vi "Section parameter check.vi"(8 "error in":errorcluster, 9 "Row number":u32, 10 "Tbl Refnum in":refnum<vi>, 11 "Tree Refnum in":refnum<vi>) -> (0 "error out":errorcluster, 1 "Check result":string="√", 2 "Tbl Refnum out":refnum<vi>, 3 "Tree Refnum out":refnum<vi>)   [LabVIEW 2010]
panel:
  out "Enum":T1(ring)=enum."float"
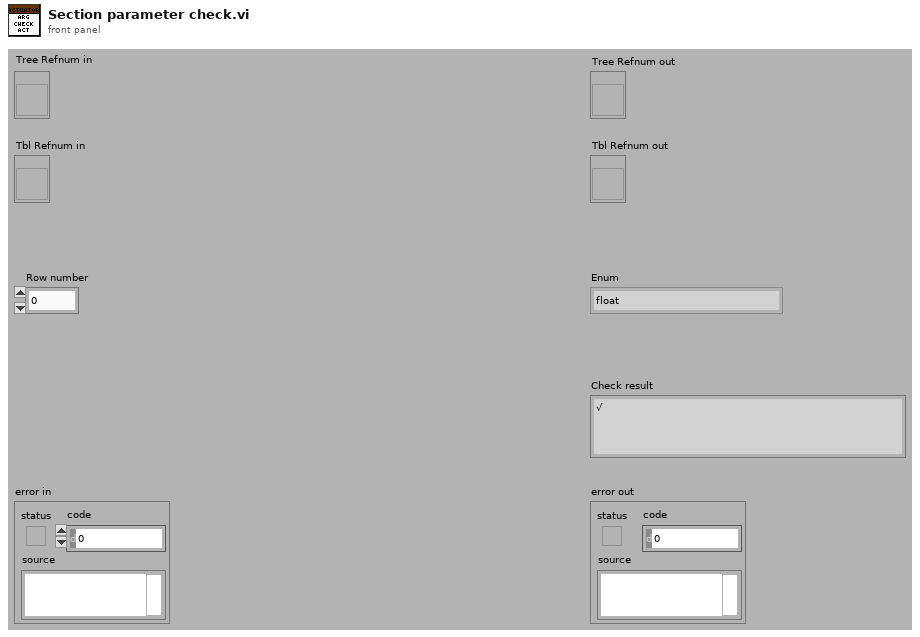
[diagram p1: front panel]
types:
  T1 = enum16{"char", "float", "double", "int", "long", "qword", "enum"}
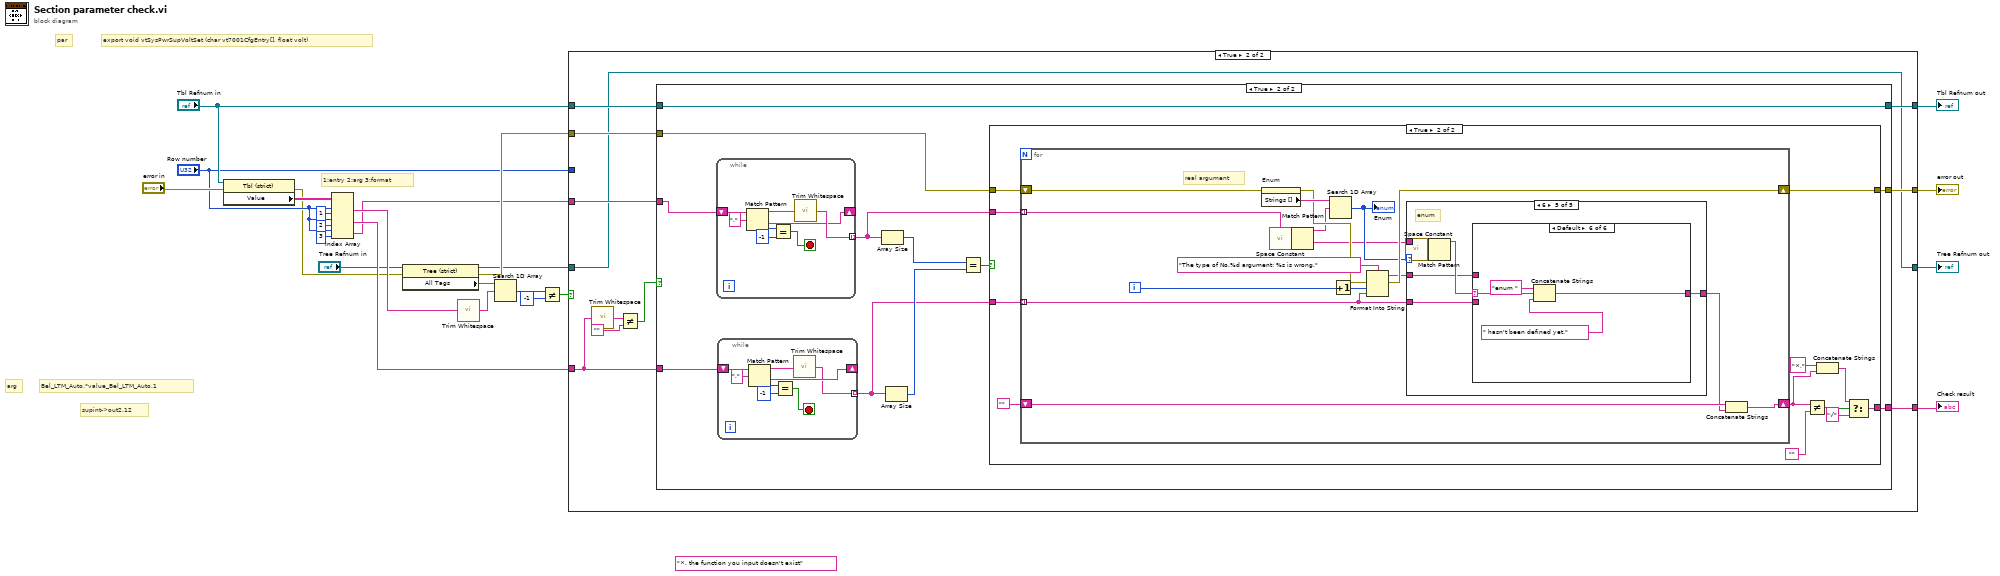
[diagram p0: block diagram]
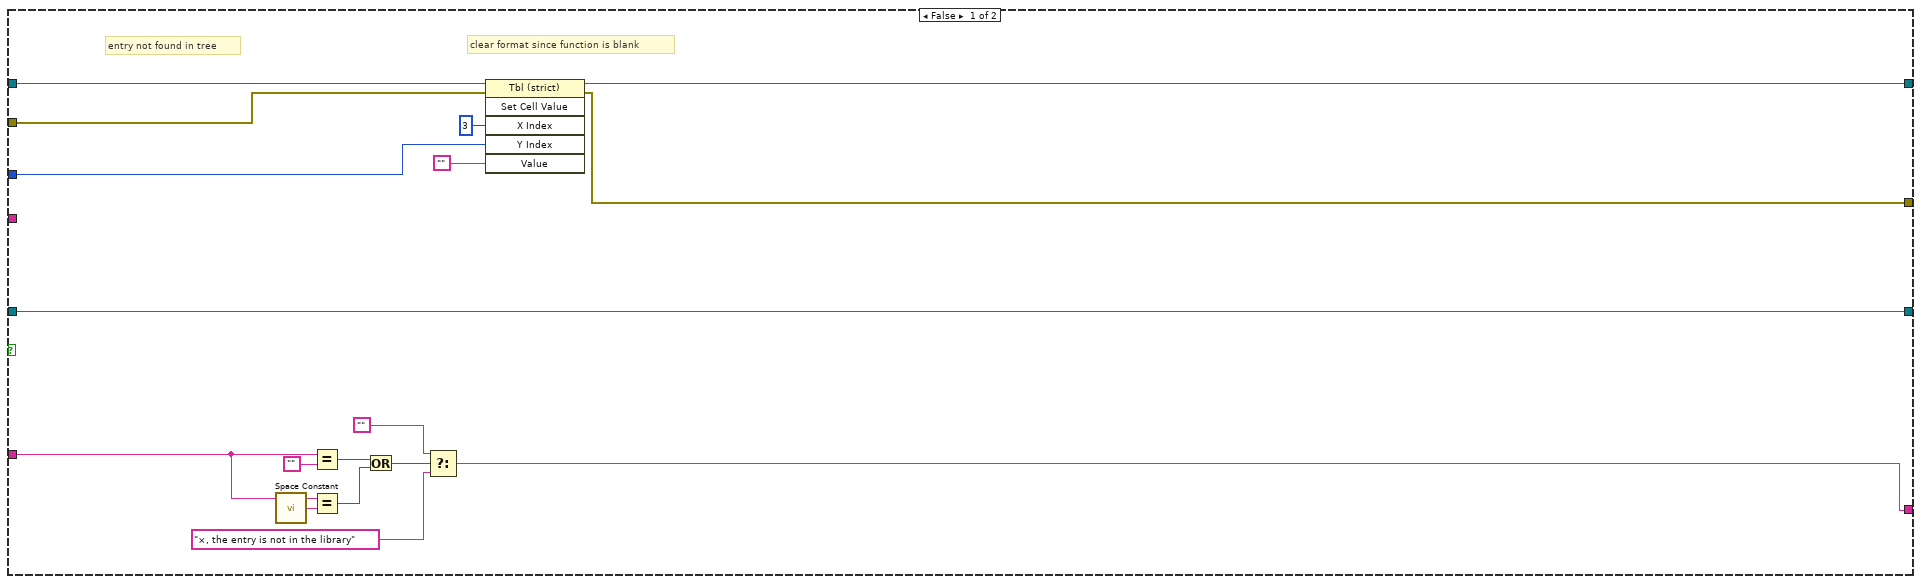
[diagram p2: hidden frame]
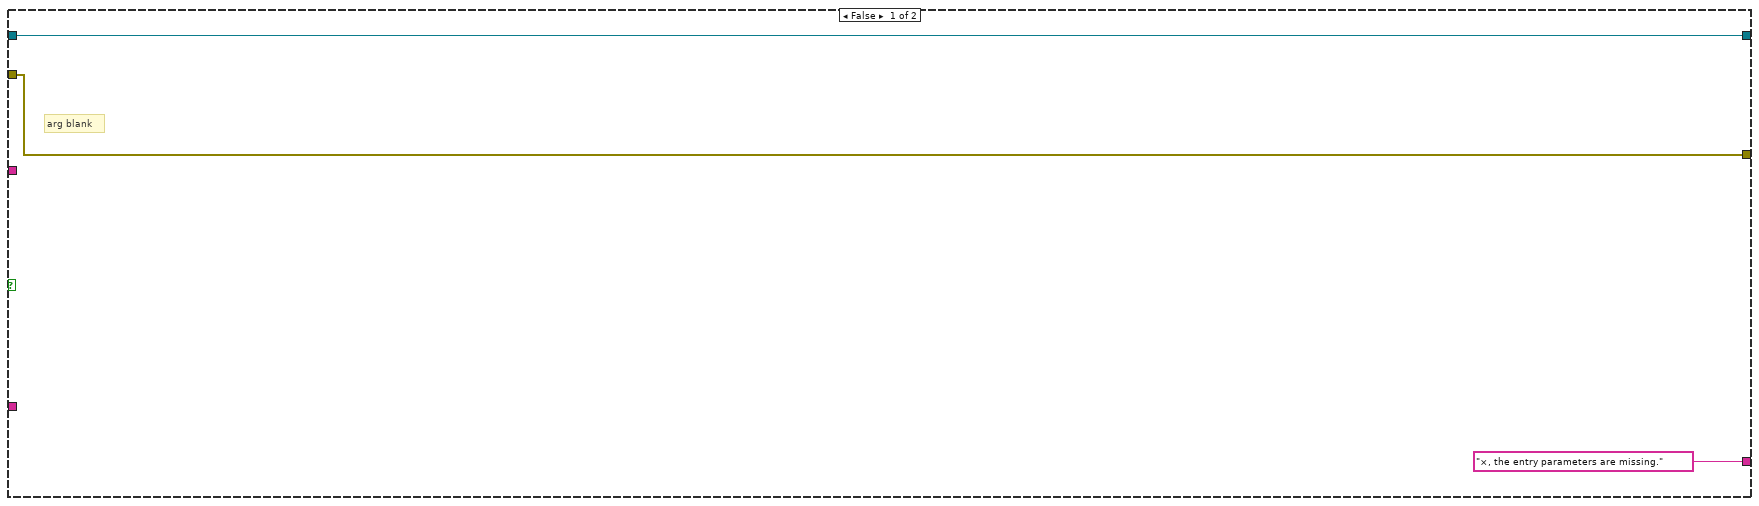
[diagram p3: hidden frame]
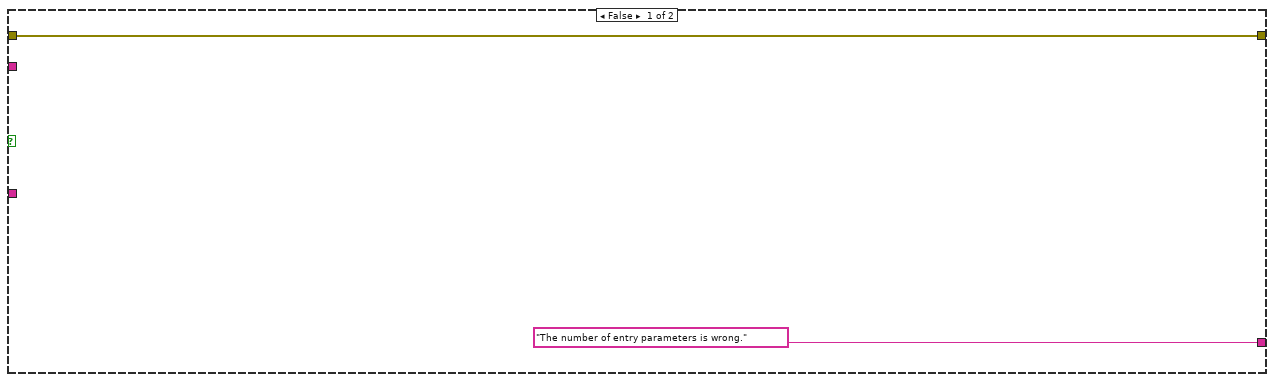
[diagram p4: hidden frame]
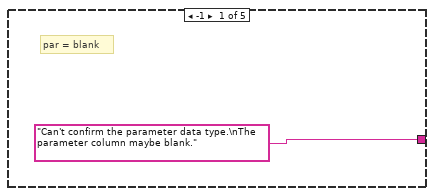
[diagram p5: hidden frame]
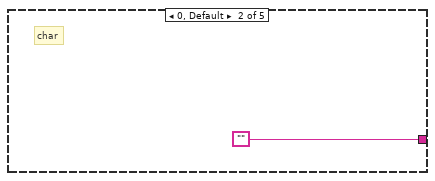
[diagram p6: hidden frame]
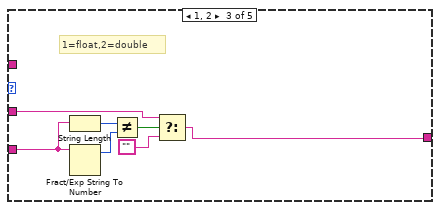
[diagram p7: hidden frame]
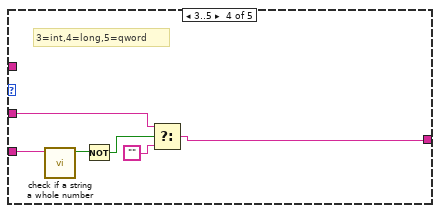
[diagram p8: hidden frame]
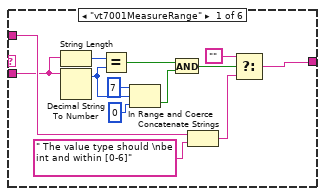
[diagram p9: hidden frame]
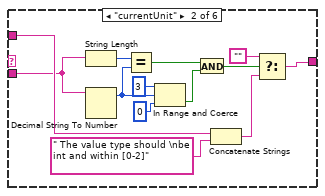
[diagram p10: hidden frame]
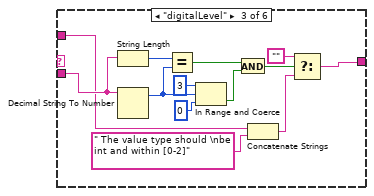
[diagram p11: hidden frame]
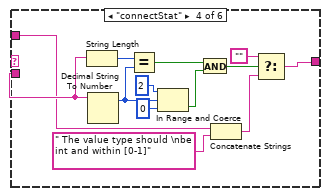
[diagram p12: hidden frame]
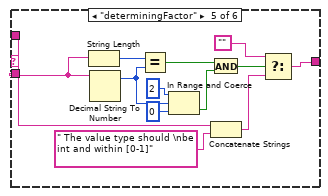
[diagram p13: hidden frame]
diagram:
  (unwired) "×, the function you input doesn't exist" ("Value")
  # "arg"
  # "par"
  # "1:entry 2:arg 3:format"
  # "Bel_LTM_Auto,*value_Bel_LTM_Auto,1"
  # "supint->out2,12"
  # "export void vtSysPwrSupVoltSet (char vt7001CfgEntry[], float volt)"
  n1 = property class="Tbl (strict)"(reference="Tbl Refnum in", error in="error in") -> (error out=w1:errorcluster, "Value"=w11:string[][])  [unwired: 1 out]
  n2 = Index Array(array=w11, index (row) #1="Row number", index (col) #1=1 ("disabled index (col)"), index (row) #2="Row number", index (col) #2=2 ("index (col)"), index (row) #3="Row number", index (col) #3=3 ("disabled index (col)")) -> (element #1=w5:string, element #2=w4:string, element #3=w3:string)
  n3 = property on="Property Node" class="Tree (strict)"(reference="Tree Refnum in", error in=w1) -> (reference out=w14:refnum<vi>, error out=w15:errorcluster, "All Tags"=w19:string[])
  n4 = call <vilib>:"Trim Whitespace.vi"("string"=w5) -> ("trimmed string"=w18:string)  [unwired: 1 in]
  n5 = Search 1D Array(1D array=w19, element=w18) -> (index of element=w17:i32)  [unwired: 1 in]
  n6 = Not Equal?(x=w17, y=-1) -> (x != y?=w23:bool)
  n7 = case shown="True" w23 {
    tunnel: w3 -> [_ w51]
    tunnel: w4 -> [w30 w42]
    tunnel: w15 -> [w33 w50]
    tunnel: [w24 w49] -> w22
    tunnel: [w37 w48] -> w21
    tunnel: "Tbl Refnum in" -> [w34 w47]
    tunnel: "Row number" -> [w35 _]
    tunnel: [w38 w46] -> w20
    tunnel: w14 -> [w36 w41]
    tunnel: [w36 w41] -> w13
    frame False {
      # "clear format since function is blank"
      # "entry not found in tree"
      n8 = call <vilib>:"Space Constant.vi"() -> ("String"=w31:string)
      n9 = Equal?(x=w30, y="") -> (x = y?=w29:bool)
      n10 = Equal?(x=w30, y=w31) -> (x = y?=w28:bool)
      n11 = Or(x=w29, y=w28) -> (x .or. y?=w27:bool)
      n12 = Select(t="", s=w27, f="×, the entry is not in the library") -> (s? t:f=w24:string)
      n13 = invoke class="Tbl (strict)" method="Set Cell Value"(reference=w34, error in=w33, "X Index"=u32 3, "Y Index"=w35, "Value"="") -> (reference out=w38:refnum<vi>, error out=w37:errorcluster)  [unwired: 1 in, 4 out]
    }
    frame True {
      n14 = call <vilib>:"Trim Whitespace.vi"("string"=w42) -> ("trimmed string"=w45:string)  [unwired: 1 in]
      n15 = Not Equal?(x=w45, y="") -> (x != y?=w43:bool)
      n16 = case shown="True" w43 {
        tunnel: w51 -> [_ w55]
        tunnel: w42 -> [_ w60]
        tunnel: w50 -> [w53 w59]
        tunnel: ["×, the entry parameters are missing." w58] -> w49
        tunnel: [w53 w57] -> w48
        tunnel: w47 -> [w54 w56]
        tunnel: [w54 w56] -> w46
        frame False {
          # "arg blank"
        }
        frame True {
          n17 = while {
            shift-right: [w195] -> _
            shift-left: w55 -> [w202]
            tunnel: [w196] -> w62 mode=indexing
            stop <- w198 stop-if-true
            n18 = Match Pattern(string=w202, regular expression=",") -> (before substring=w197:string, after substring=w195:string, offset past match=w200:i32)  [unwired: 1 in, 1 out]
            n19 = Equal?(x=w200, y=-1) -> (x = y?=w198:bool)
            n20 = call <vilib>:"Trim Whitespace.vi"("string"=w197) -> ("trimmed string"=w196:string)  [unwired: 1 in]
          }
          n21 = while {
            shift-right: [w190] -> _
            shift-left: w60 -> [w194]
            tunnel: [w187] -> w61 mode=indexing
            stop <- w189 stop-if-true
            n22 = Match Pattern(string=w194, regular expression=",") -> (before substring=w188:string, after substring=w190:string, offset past match=w192:i32)  [unwired: 1 in, 1 out]
            n23 = Equal?(x=w192, y=-1) -> (x = y?=w189:bool)
            n24 = call <vilib>:"Trim Whitespace.vi"("string"=w188) -> ("trimmed string"=w187:string)  [unwired: 1 in]
          }
          n25 = Array Size(array=w62) -> (size(s)=w65:i32)
          n26 = Array Size(array=w61) -> (size(s)=w64:i32)
          n27 = Equal?(x=w65, y=w64) -> (x = y?=w63:bool)
          n28 = case shown="True" w63 {
            tunnel: w62 -> [_ w79]
            tunnel: w61 -> [_ w78]
            tunnel: ["The number of entry parameters is wrong." w73] -> w58
            tunnel: w59 -> [w66 w72]
            tunnel: [w66 w71] -> w57
            frame False {
            }
            frame True {
              n29 = for {
                tunnel: w79 -> [w80] mode=indexing
                tunnel: w78 -> [w91] mode=indexing
                shift-right: [w95] -> w69
                shift-left: "" -> [w96]
                shift-right: [w93] -> w71
                shift-left: w72 -> [w94]
                i -> [w92]
                # "real argument"
                n30 = property on="Enum" class="Enum (strict)"(error in=w94) -> (error out=w85:errorcluster, "Strings []"=w89:string[])  [unwired: 1 in, 1 out]
                n31 = call <vilib>:"Space Constant.vi"() -> ("String"=w90:string)
                n32 = Match Pattern(string=w80, regular expression=w90) -> (before substring=w82:string, after substring=w81:string)  [unwired: 1 in, 2 out]
                n33 = Search 1D Array(1D array=w89, element=w82) -> (index of element=w88:i32)  [unwired: 1 in]
                "Enum" <- w88
                n34 = Increment(x=w92) -> (x+1=w86:i32)
                n35 = Format Into String(format string="The type of No.%d argument: %s is wrong.", error in=w85, w86, w91) -> (resulting string=w84:string, error out=w93:errorcluster)  [unwired: 1 in]
                n36 = case shown="6" w88 {
                  tunnel: w91 -> [_ _ w103 w108 w113]
                  tunnel: w84 -> [_ _ w100 w111 w114]
                  tunnel: ["Can't confirm the parameter data type.\nThe parameter column maybe blank." "" w99 w109 w112] -> w83
                  tunnel: w81 -> [_ _ _ _ w117]
                  frame -1 {
                    # "par = blank"
                  }
                  frame 0, Default {
                    # "char"
                  }
                  frame 1, 2 {
                    # "1=float,2=double"
                    n37 = String Length(string=w103) -> (length=w105:i32)
                    n38 = Fract/Exp String To Number(string=w103) -> (offset past number=w104:i32)  [unwired: 3 in, 1 out]
                    n39 = Not Equal?(x=w105, y=w104) -> (x != y?=w102:bool)
                    n40 = Select(t=w100, s=w102, f="") -> (s? t:f=w99:string)
                  }
                  frame 3..5 {
                    # "3=int,4=long,5=qword"
                    n41 = call "check if a string a whole number.vi"("input string"=w108) -> ("is a whole number?"=w107:bool)  [unwired: 10 in]
                    n42 = Not(x=w107) -> (.not. x?=w106:bool)
                    n43 = Select(t=w111, s=w106, f="") -> (s? t:f=w109:string)
                  }
                  frame 6 {
                    # "enum"
                    n44 = call <vilib>:"Space Constant.vi"() -> ("String"=w116:string)
                    n45 = Match Pattern(string=w117, regular expression=w116) -> (before substring=w115:string)  [unwired: 1 in, 3 out]
                    n46 = case shown="Default" w115 {
                      selector: w115 -> [_ _ _ _ _ w186]
                      tunnel: w114 -> [w120 w133 w145 w158 w171 _]
                      tunnel: w113 -> [w119 w132 w146 w159 w173 _]
                      tunnel: [w118 w131 w144 w157 w172 w184] -> w112
                      frame "vt7001MeasureRange" {
                        n47 = String Length(string=w119) -> (length=w130:i32)
                        n48 = Decimal String To Number(string=w119) -> (offset past number=w128:i32)  [unwired: 2 in, 1 out]
                        n49 = Equal?(x=w130, y=w128) -> (x = y?=w129:bool)
                        n50 = In Range and Coerce(upper limit=7, x=w128, lower limit=0) -> (In Range?=w125:bool)  [unwired: 1 out]
                        n51 = And(x=w129, y=w125) -> (x .and. y?=w124:bool)
                        n52 = Concatenate Strings(w120, " The value type should \nbe int and within [0-6]" ("string")) -> (w122:string)
                        n53 = Select(t="", s=w124, f=w122) -> (s? t:f=w118:string)
                      }
                      frame "currentUnit" {
                        n54 = String Length(string=w132) -> (length=w143:i32)
                        n55 = Decimal String To Number(string=w132) -> (offset past number=w141:i32)  [unwired: 2 in, 1 out]
                        n56 = Equal?(x=w143, y=w141) -> (x = y?=w142:bool)
                        n57 = In Range and Coerce(upper limit=3, x=w141, lower limit=0) -> (In Range?=w138:bool)  [unwired: 1 out]
                        n58 = And(x=w142, y=w138) -> (x .and. y?=w137:bool)
                        n59 = Concatenate Strings(w133, " The value type should \nbe int and within [0-2]" ("string")) -> (w135:string)
                        n60 = Select(t="", s=w137, f=w135) -> (s? t:f=w131:string)
                      }
                      frame "digitalLevel" {
                        n61 = String Length(string=w146) -> (length=w156:i32)
                        n62 = Decimal String To Number(string=w146) -> (offset past number=w154:i32)  [unwired: 2 in, 1 out]
                        n63 = Equal?(x=w156, y=w154) -> (x = y?=w155:bool)
                        n64 = In Range and Coerce(upper limit=3, x=w154, lower limit=0) -> (In Range?=w151:bool)  [unwired: 1 out]
                        n65 = And(x=w155, y=w151) -> (x .and. y?=w150:bool)
                        n66 = Concatenate Strings(w145, " The value type should \nbe int and within [0-2]" ("string")) -> (w148:string)
                        n67 = Select(t="", s=w150, f=w148) -> (s? t:f=w144:string)
                      }
                      frame "connectStat" {
                        n68 = String Length(string=w159) -> (length=w169:i32)
                        n69 = Decimal String To Number(string=w159) -> (offset past number=w167:i32)  [unwired: 2 in, 1 out]
                        n70 = Equal?(x=w169, y=w167) -> (x = y?=w168:bool)
                        n71 = In Range and Coerce(upper limit=2, x=w167, lower limit=0) -> (In Range?=w164:bool)  [unwired: 1 out]
                        n72 = And(x=w168, y=w164) -> (x .and. y?=w163:bool)
                        n73 = Concatenate Strings(w158, " The value type should \nbe int and within [0-1]" ("string")) -> (w161:string)
                        n74 = Select(t="", s=w163, f=w161) -> (s? t:f=w157:string)
                      }
                      frame "determiningFactor" {
                        n75 = String Length(string=w173) -> (length=w182:i32)
                        n76 = Decimal String To Number(string=w173) -> (offset past number=w180:i32)  [unwired: 2 in, 1 out]
                        n77 = Equal?(x=w182, y=w180) -> (x = y?=w181:bool)
                        n78 = In Range and Coerce(upper limit=2, x=w180, lower limit=0) -> (In Range?=w177:bool)  [unwired: 1 out]
                        n79 = And(x=w181, y=w177) -> (x .and. y?=w176:bool)
                        n80 = Concatenate Strings(w171, " The value type should \nbe int and within [0-1]" ("string")) -> (w170:string)
                        n81 = Select(t="", s=w176, f=w170) -> (s? t:f=w172:string)
                      }
                      frame Default {
                        n82 = Concatenate Strings("enum " ("string"), w186, " hasn't been defined yet.") -> (w184:string)
                      }
                    }
                  }
                }
                n83 = Concatenate Strings(w96, w83) -> (w95:string)
              }
              n84 = Not Equal?(x=w69, y="") -> (x != y?=w75:bool)
              n85 = Concatenate Strings("×,", w69) -> (w68:string)
              n86 = Select(t=w68, s=w75, f="√") -> (s? t:f=w73:string)
            }
          }
        }
      }
    }
  }
  "Check result" <- w22
  "error out" <- w21
  "Tbl Refnum out" <- w20
  "Tree Refnum out" <- w13
